vi "Write Odometry Position Variable.vi"(6 "wheel angles":dbl[](array[numeric]), 8 "theta'":dbl, 9 "x', y'":dbl[](array[numeric]), 10 "theta":dbl, 11 "x,y":dbl[](array[numeric])) -> ()   [LabVIEW 2011]
uses:
  <vilib>/Analysis/coordinate.llb/2D Cartesian Coordinate Rotation (Scalar).vi
  <vilib>/Analysis/NI_AALPro.lvlib
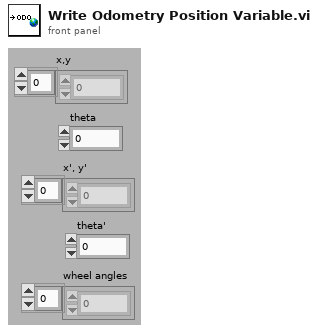
[diagram p1: front panel]
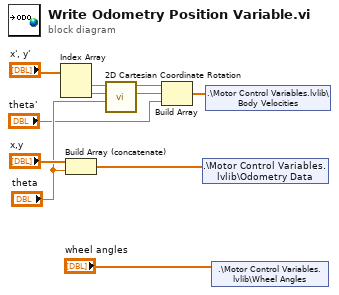
[diagram p0: block diagram]
diagram:
  n1 = Index Array(array="x', y'") -> (element #1=w8:dbl, element #2=w7:dbl)  [unwired: 2 in]
  n2 = Build Array (concatenate)("x,y", "theta") -> (w10:dbl[])
  n3 = call-poly <vilib>:"2D Cartesian Coordinate Rotation.vi"("theta"="theta", "y"=w7, "x"=w8) -> ("y out"=w4:dbl, "x out"=w5:dbl)  [unwired: 7 out]
  n4 = Build Array(w5, w4, "theta'") -> (w2:dbl[])
  n5 = shared-variable ".\\Motor Control Variables.lvlib\\Odometry Data"(w10) -> ()  [unwired: 1 in, 1 out]
  n6 = shared-variable ".\\Motor Control Variables.lvlib\\Body Velocities"(w2) -> ()  [unwired: 1 in, 1 out]
  n7 = shared-variable ".\\Motor Control Variables.lvlib\\Wheel Angles"("wheel angles") -> ()  [unwired: 1 in, 1 out]
